vi "Compare Calls.vi"(8 "error in (no error)":errorcluster, 9 "VI Call 2":refnum<class "VI Call.lvclass">, 10 "VI Call 1":refnum<class "VI Call.lvclass">, 11 "Tolerant Numeric Comparator In":refnum<class "Tolerant Numeric Input Comparator.lvclass">) -> (0 "error out":errorcluster, 1 "Description":string, 2 "Equal?":bool)   [LabVIEW 2020, in "Tolerant Numeric Input Comparator.lvclass"]
uses:
  Tolerant Numeric Input Comparator.lvclass
  Core/VI Call/VI Call.lvclass
  Tolerant Numeric Input Comparator.lvclass/Tolerant Numeric Input Comparator.ctl
  Core/Comparator/Describe Variant.vi
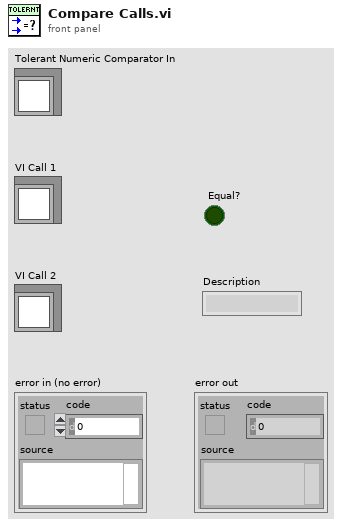
[diagram p1: front panel]
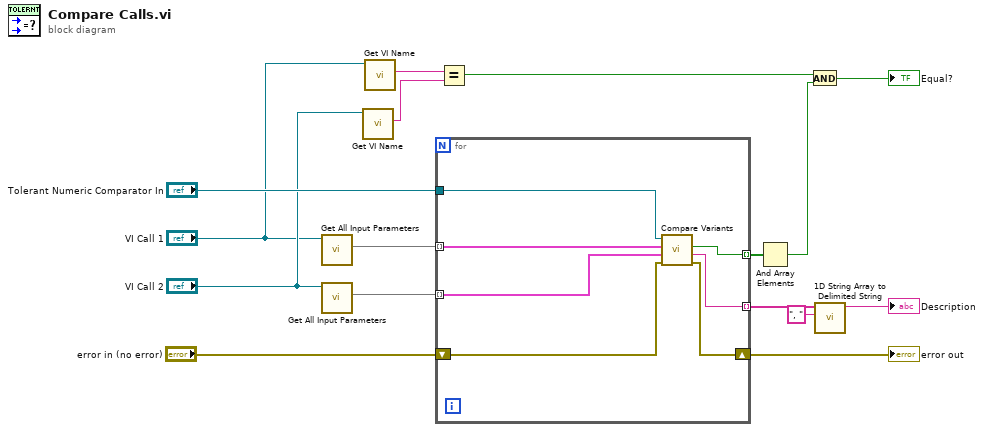
[diagram p0: block diagram]
diagram:
  n1 = call-dynamic "Get All Input Parameters.vi"("VI Call in"="VI Call 1") -> ("Input Parameters"=w16:map{string, variant})  [unwired: 9 in, 1 out]
  n2 = call-dynamic "Get All Input Parameters.vi"("VI Call in"="VI Call 2") -> ("Input Parameters"=w15:map{string, variant})  [unwired: 9 in, 1 out]
  n3 = call-dynamic "Get VI Name.vi"("VI Call In"="VI Call 2") -> ("VI Name"=w4:string)  [unwired: 9 in, 1 out]
  n4 = call-dynamic "Get VI Name.vi"("VI Call In"="VI Call 1") -> ("VI Name"=w5:string)  [unwired: 9 in, 1 out]
  n5 = for {
    tunnel: w16 -> [w23] mode=indexing
    tunnel: w15 -> [w22] mode=indexing
    tunnel: "Tolerant Numeric Comparator In" -> [w21]
    tunnel: [w20] -> w13 mode=indexing
    shift-right: [w18] -> w11
    shift-left: "error in (no error)" -> [w19]
    tunnel: [w17] -> w3 mode=indexing
    n6 = call "Compare Variants.vi"("error in (no error)"=w19, "Parameter 2"=w22, "Parameter 1"=w23, "Tolerant Numeric Comparator In"=w21) -> ("error out"=w18:errorcluster, "Description"=w17:string, "Equal?"=w20:bool)  [unwired: 5 in]
  }
  "error out" <- w11
  n7 = Equal?(x=w5, y=w4) -> (x = y?=w10:bool)
  n8 = And Array Elements(Boolean array=w13) -> (logical AND=w7:bool)
  n9 = And(x=w10, y=w7) -> (x .and. y?=→"Equal?":bool)
  n10 = call <vilib>:"1D String Array to Delimited String.vi"("delimiter"=", ", "string array"=w3) -> ("delimited string"=→"Description":string)  [unwired: 9 in]
